vi "ofdm_mes_ce.vi"(11 "ZF \nchannel \nestimates":cdb[](array[numeric])) -> (3 "interpolated\n mes carrier CE":cdb[](array[numeric]))   [LabVIEW 2014]
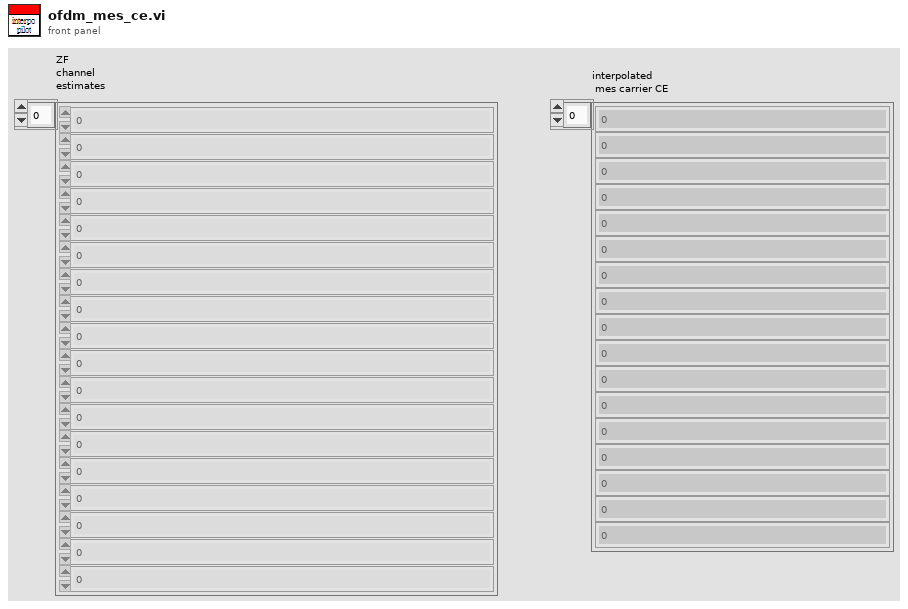
[diagram p1: front panel]
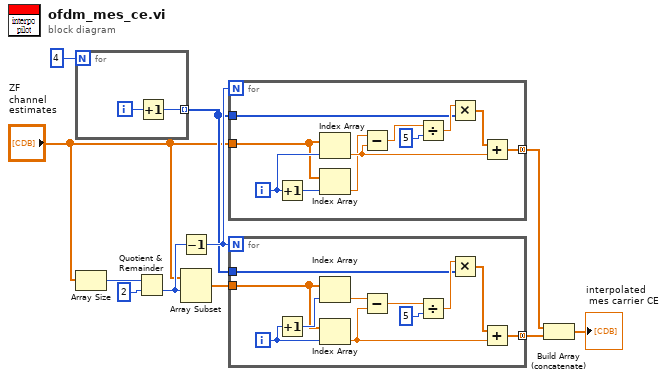
[diagram p0: block diagram]
diagram:
  n1 = for {
    N: 4 -> [_]
    tunnel: [w12] -> w6 mode=indexing
    i -> [w13]
    n2 = Increment(x=w13) -> (x+1=w12:i32)
  }
  n3 = Array Size(array="ZF \nchannel \nestimates") -> (size(s)=w11:i32)
  n4 = Quotient & Remainder(x=w11, y=2) -> (floor(x/y)=w9:i32)  [unwired: 1 out]
  n5 = Decrement(x=w9) -> (x-1=w8:i32)
  n6 = Array Subset(array="ZF \nchannel \nestimates", index=w9) -> (w3:cdb[])  [unwired: 1 in]
  n7 = for {
    N: w8 -> [_]
    tunnel: "ZF \nchannel \nestimates" -> [w22]
    tunnel: w6 -> [w18]
    tunnel: [w16] -> w4 mode=concatenating
    i -> [w23]
    n8 = Increment(x=w23) -> (x+1=w24:i32)
    n9 = Index Array(array=w22, index=w23) -> (element=w15:cdb)
    n10 = Index Array(array=w22, index=w24) -> (element=w14:cdb)
    n11 = Subtract(x=w14, y=w15) -> (x-y=w21:cdb)
    n12 = Divide(x=w21, y=5) -> (x/y=w19:cdb)
    n13 = Multiply(x=w19, y=w18) -> (x*y=w17:cdb[])
    n14 = Add(x=w17, y=w15) -> (x+y=w16:cdb[])
  }
  n15 = for {
    N: w8 -> [_]
    tunnel: w3 -> [w30]
    tunnel: w6 -> [w28]
    tunnel: [w27] -> w2 mode=concatenating
    i -> [w29]
    n16 = Increment(x=w29) -> (x+1=w31:i32)
    n17 = Index Array(array=w30, index=w31) -> (element=w26:cdb)
    n18 = Index Array(array=w30, index=w29) -> (element=w25:cdb)
    n19 = Subtract(x=w26, y=w25) -> (x-y=w32:cdb)
    n20 = Divide(x=w32, y=5) -> (x/y=w34:cdb)
    n21 = Multiply(x=w34, y=w28) -> (x*y=w35:cdb[])
    n22 = Add(x=w35, y=w25) -> (x+y=w27:cdb[])
  }
  n23 = Build Array (concatenate)(w4, w2) -> (→"interpolated\n mes carrier CE":cdb[])
